vi "Digital Trigger Control.vi"(0 "Operation":T1(ring)) -> (15 "error out":errorcluster)   [LabVIEW 2019]
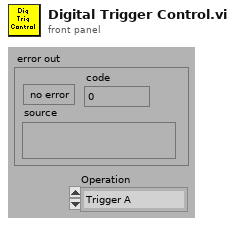
[diagram p1: front panel]
types:
  T1 = enum16{"Trigger A", "Trigger B", "Clear Triggers"}
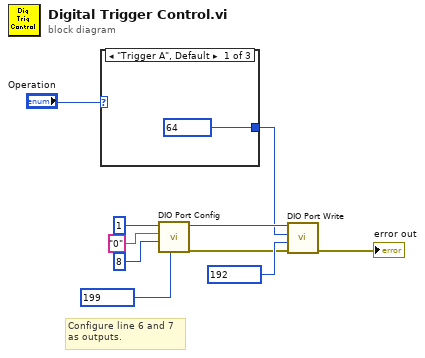
[diagram p0: block diagram]
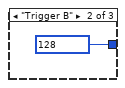
[diagram p2: hidden frame]
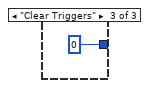
[diagram p3: hidden frame]
diagram:
  # "Configure line 6 and 7\nas outputs."
  n1 = case shown="\"Trigger A\", Default" "Operation" {
    tunnel: [64 ("line direction map") 128 ("line direction map") 0 ("line direction map")] -> w5
    frame "Trigger A", Default {
    }
    frame "Trigger B" {
    }
    frame "Clear Triggers" {
    }
  }
  n2 = call "DIO Port Config.vi"("line direction map"=199, "port width"=i16 8, "digital channel"="0", "device"=i16 1) -> ("error out"=w2:errorcluster, "task ID out"=w6:u32)  [unwired: 6 in]
  n3 = call "DIO Port Write.vi"("error in (no error)"=w2, "line mask"=192 ("line direction map"), "pattern"=w5, "task ID"=w6) -> ("error out"=→"error out":errorcluster)  [unwired: 6 in, 1 out]
